vi "Get Application Information.vi"(8 "error out":errorcluster, 11 "Build Name":string="LabActor") -> (0 "Error Out":errorcluster, 1 "Last modified":string, 2 "Build version":string, 3 "Path":path, 4 "Build Specification Version":T1)   [LabVIEW 2016]
uses:
  <vilib>/AppBuilder/AB_API_Simple/Build Specification Version.ctl
  <vilib>/AppBuilder/AB_API_Simple/Get Build Specification Version (path).vi
  <vilib>/AppBuilder/AB_API_Simple/NI_App_Builder_API.lvlib
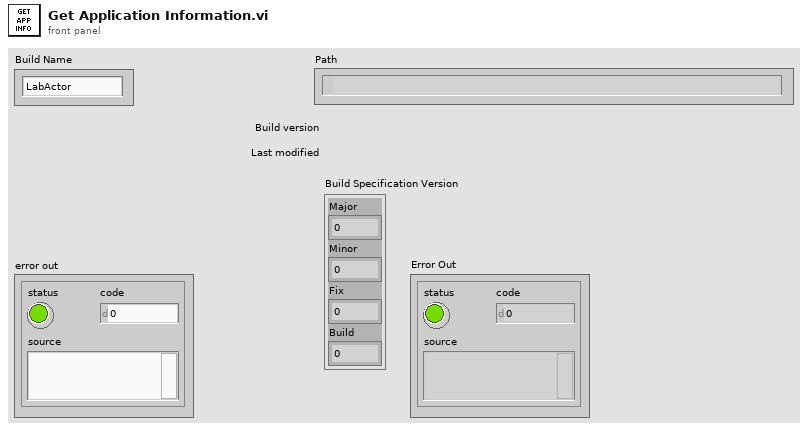
[diagram p1: front panel]
types:
  T1 = typedef "NI_App_Builder_API.lvlib/Build Specification Version.ctl" = cluster{"Major":u16, "Minor":u16, "Fix":u16, "Build":u16}
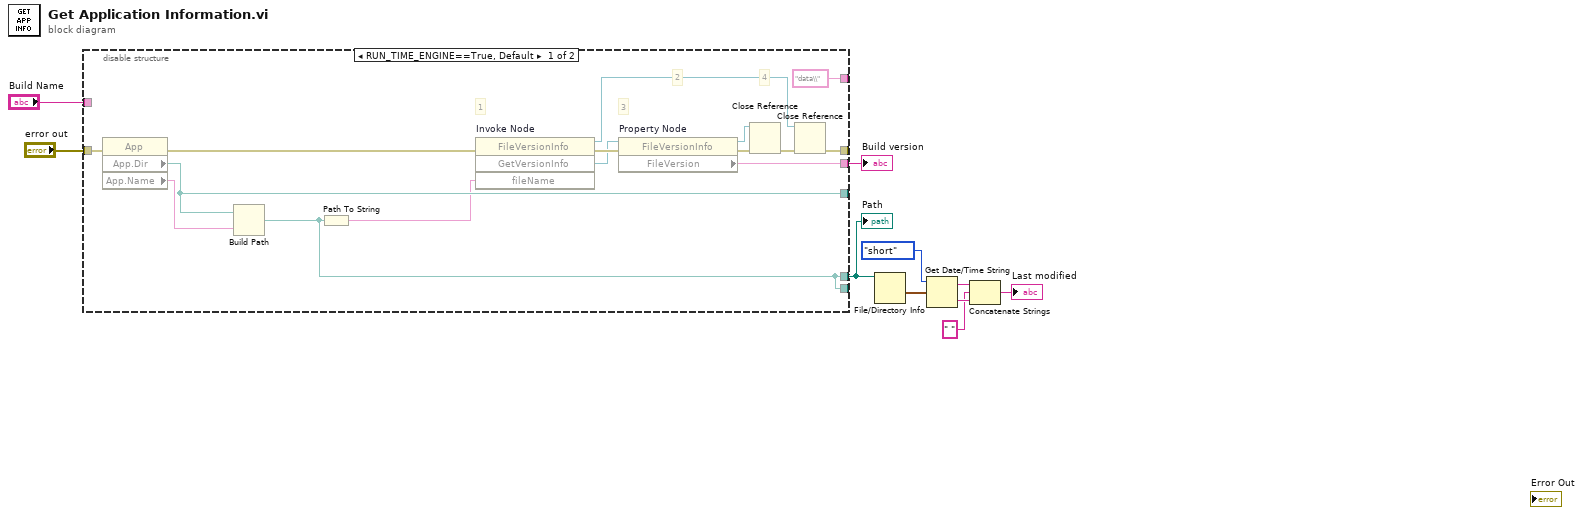
[diagram p0: block diagram]
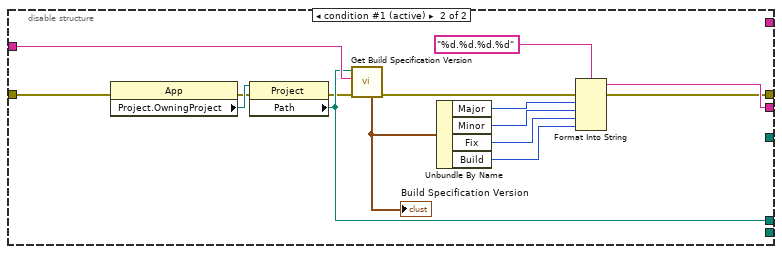
[diagram p2: hidden frame]
diagram:
  n1 = disable-structure shown="RUN_TIME_ENGINE==True, Default" {
    disable-tunnel: [w24 _] -> _
    disable-tunnel: "error out" -> [w23 w26]
    disable-tunnel: [w13 w30] -> _
    disable-tunnel: [w12 _] -> _
    disable-tunnel: ["data\\" ("string") _] -> _
    disable-tunnel: "Build Name" -> [_ w39]
    disable-tunnel: [w12 w38] -> w2
    disable-tunnel: [w11 w32] -> w1
    frame condition #0 {
      # "4"
      # "3"
      # "2"
      # "1"
      n2 = property class="App"(error in=w23) -> (error out=w14:errorcluster, "App.Dir"=w24:path, "App.Name"=w25:string)  [unwired: 1 in, 1 out]
      n3 = Build Path(base path=w24, name or relative path=w25) -> (appended path=w12:path)
      n4 = Path To String(path=w12) -> (string=w15:string)
      n5 = invoke on="Invoke Node" class="FileVersionInfo" method="GetVersionInfo"(error in=w14, "fileName"=w15) -> (reference out=w21:refnum<k24>, error out=w17:errorcluster, "GetVersionInfo"=w16:refnum<k24>)  [unwired: 2 in, 1 out]
      n6 = property on="Property Node" class="FileVersionInfo"(reference=w16, error in=w17) -> (reference out=w18:refnum<k24>, error out=w19:errorcluster, "FileVersion"=w11:string)
      n7 = Close Reference(reference=w18, error in (no error)=w19) -> (error out=w20:errorcluster)
      n8 = Close Reference(reference=w21, error in (no error)=w20) -> (error out=w13:errorcluster)
    }
    frame condition #1 (active) {
      n9 = property class="App"(error in=w26) -> (error out=w27:errorcluster, "Project.OwningProject"=w40:refnum<vi>)  [unwired: 1 in, 1 out]
      n10 = property class="Project"(reference=w40, error in=w27) -> (error out=w28:errorcluster, "Path"=w38:path)  [unwired: 1 out]
      n11 = call-poly <vilib>:"Get Build Specification Version.vi"("error in (no error)"=w28, "Name of build specification"=w39, "Path to project"=w38) -> ("error out"=w29:errorcluster, "Build Specification Version"=w31:T1)  [unwired: 7 in]
      "Build Specification Version" <- w31
      n12 = Unbundle By Name(w31) -> ("Major"=w37:u16, "Minor"=w36:u16, "Fix"=w35:u16, "Build"=w34:u16)
      n13 = Format Into String(format string="%d.%d.%d.%d", error in=w29, w37, w36, w35, w34) -> (resulting string=w32:string, error out=w30:errorcluster)  [unwired: 1 in]
    }
  }
  "Path" <- w2
  "Build version" <- w1
  n14 = File/Directory Info(path=w2) -> (last mod=w4:timestamp)  [unwired: 1 in, 6 out]
  n15 = Get Date/Time String(date format (0)=enum16{"short", "long", "abbreviated"}."short", seconds (now)=w4) -> (date string=w6:string, time string=w7:string)  [unwired: 1 in]
  n16 = Concatenate Strings(w6, " " ("string"), w7) -> (→"Last modified":string)
